vi "QueryServer_GetRequest_Invoke.vi"(6 "error in (no error)":errorcluster, 9 "gRPCid":T1) -> (0 "error out":errorcluster, 1 "parameter":string, 2 "command":string, 3 "gRPCid out":T1)   [LabVIEW 2019, in "labview-grpc-query-server.lvlib"]
uses:
  labview-grpc-query-server.lvlib
  QueryServer_gRPCid.ctl
  QueryServer_InvokeRequest.ctl
  build/Debug/labview_grpc_server.dll
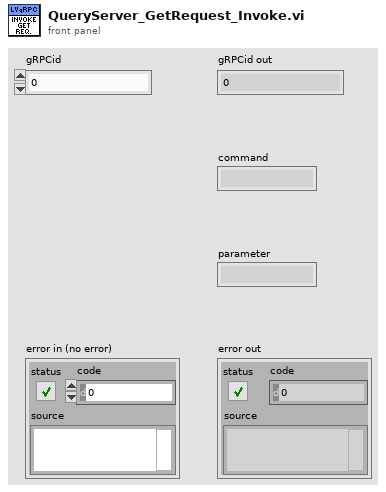
[diagram p1: front panel]
types:
  T1 = typedef "labview-grpc-query-server.lvlib/QueryServer_gRPCid.ctl" = u64
  T2 = typedef "labview-grpc-query-server.lvlib/QueryServer_InvokeRequest.ctl" = cluster{"command":string, "parameter":string}
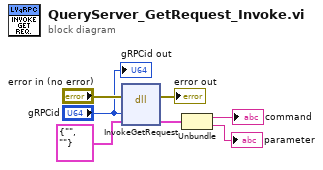
[diagram p0: block diagram]
diagram:
  n1 = dll-call lib="C:/dev/labview-grpc-server/build/Debug/labview_grpc_server.dll" fn="InvokeGetRequest"(error in="error in (no error)", "id"="gRPCid", "data"=T2 {"command"="", "parameter"=""} ("InvokeRequest")) -> (error out=→"error out":errorcluster, "data"=w3:T2)  [unwired: 4 in, 1 out]
  n2 = Unbundle(w3) -> ("command"=→"command":string, "parameter"=→"parameter":string)
  "gRPCid out" <- "gRPCid"
